vi "Intensity Graph to XY Graph (Vertical) (by ref).vi"(8 "error in (no error)":errorcluster, 11 "graph_utilities in":refnum<class "graph_utilities.lvclass">) -> (0 "error out":errorcluster, 3 "graph_utilities out":refnum<class "graph_utilities.lvclass">)   [LabVIEW 2019, in "graph_utilities.lvclass"]
doc: "Converts an Intensity Graph into a sequence of plots on a XY Graph.\n\nThe x-axis of the XY Graph will be equal to the y-axis of the Intensity Graph."
uses:
  graph_utilities.lvclass
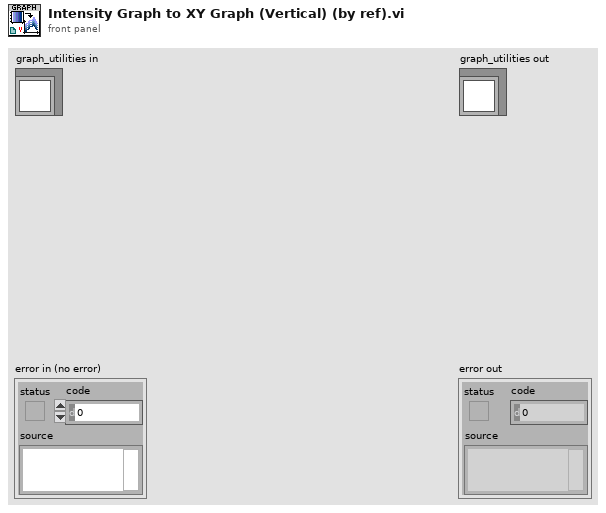
[diagram p1: front panel]
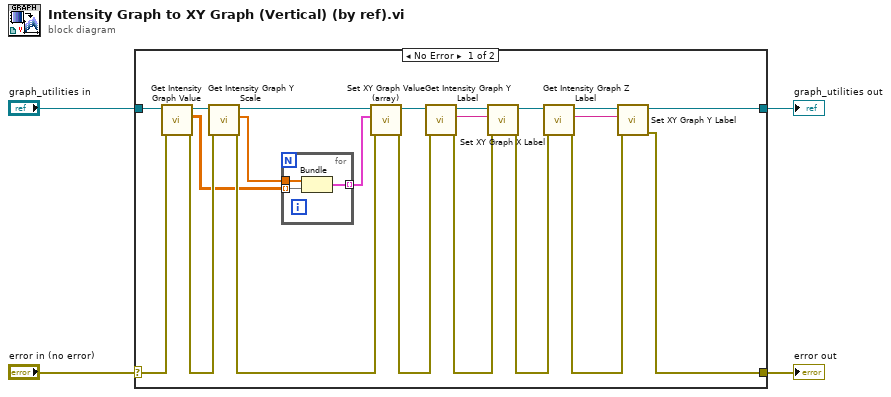
[diagram p0: block diagram]
diagram:
  n1 = case shown="No Error" "error in (no error)" {
    selector: "error in (no error)" -> [w9 w30]
    tunnel: [w6 w30] -> w3
    tunnel: [w7 w29] -> w1
    tunnel: "graph_utilities in" -> [w25 w29]
    frame No Error {
      n2 = call "Get Intensity Graph Value.vi"("error in (no error)"=w9, "graph_utilities in"=w25) -> ("error out"=w8:errorcluster, "Value"=w5:dbl[][], "graph_utilities out"=w10:refnum<class "graph_utilities.lvclass">)  [unwired: 7 in]
      n3 = call "Get Intensity Graph Y Scale.vi"("error in (no error)"=w8, "graph_utilities in"=w10) -> ("error out"=w21:errorcluster, "Y Scale"=w24:dbl[], "graph_utilities out"=w22:refnum<class "graph_utilities.lvclass">)  [unwired: 6 in, 1 out]
      n4 = for {
        tunnel: w5 -> [w27] mode=indexing
        tunnel: w24 -> [w28]
        tunnel: [w26] -> w23 mode=indexing
        n5 = Bundle("Y Scale"=w28, "Value"=w27) -> (w26:cluster{"Y Scale":dbl[], "Value":dbl[]})  [unwired: 1 in]
      }
      n6 = call "Set XY Graph Value (array).vi"("error in (no error)"=w21, "XY-data"=w23, "graph_utilities in"=w22) -> ("error out"=w13:errorcluster, "graph_utilities out"=w14:refnum<class "graph_utilities.lvclass">)  [unwired: 7 in]
      n7 = call "Get Intensity Graph Y Label.vi"("error in (no error)"=w13, "graph_utilities in"=w14) -> ("error out"=w12:errorcluster, "Y Label"=w20:string, "graph_utilities out"=w15:refnum<class "graph_utilities.lvclass">)  [unwired: 7 in]
      n8 = call "Set XY Graph X Label.vi"("error in (no error)"=w12, "X Label"=w20, "graph_utilities in"=w15) -> ("error out"=w16:errorcluster, "graph_utilities out"=w17:refnum<class "graph_utilities.lvclass">)  [unwired: 7 in]
      n9 = call "Get Intensity Graph Z Label.vi"("error in (no error)"=w16, "graph_utilities in"=w17) -> ("error out"=w11:errorcluster, "Z Label"=w19:string, "graph_utilities out"=w18:refnum<class "graph_utilities.lvclass">)  [unwired: 7 in]
      n10 = call "Set XY Graph Y Label.vi"("error in (no error)"=w11, "Y Label"=w19, "graph_utilities in"=w18) -> ("error out"=w6:errorcluster, "graph_utilities out"=w7:refnum<class "graph_utilities.lvclass">)  [unwired: 7 in]
    }
    frame Error {
    }
  }
  "error out" <- w3
  "graph_utilities out" <- w1
